vi "ArmPositionControl.vi"(9 "DriverJoystickButtons":bool[](array[boolean]), 10 "ButtonBox2":bool[](array[boolean]), 11 "Buttons":bool[](array[boolean])=[FALSE, FALSE, FALSE, FALSE, FALSE, FALSE, FALSE, FALSE, FALSE, FALSE, FALSE, FALSE]) -> ()   [LabVIEW 2015]
uses:
  Utilities/MotorPositionGlobals.vi
  Utilities/VisionGlobals.vi
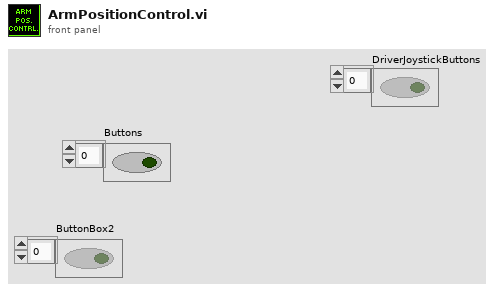
[diagram p1: front panel]
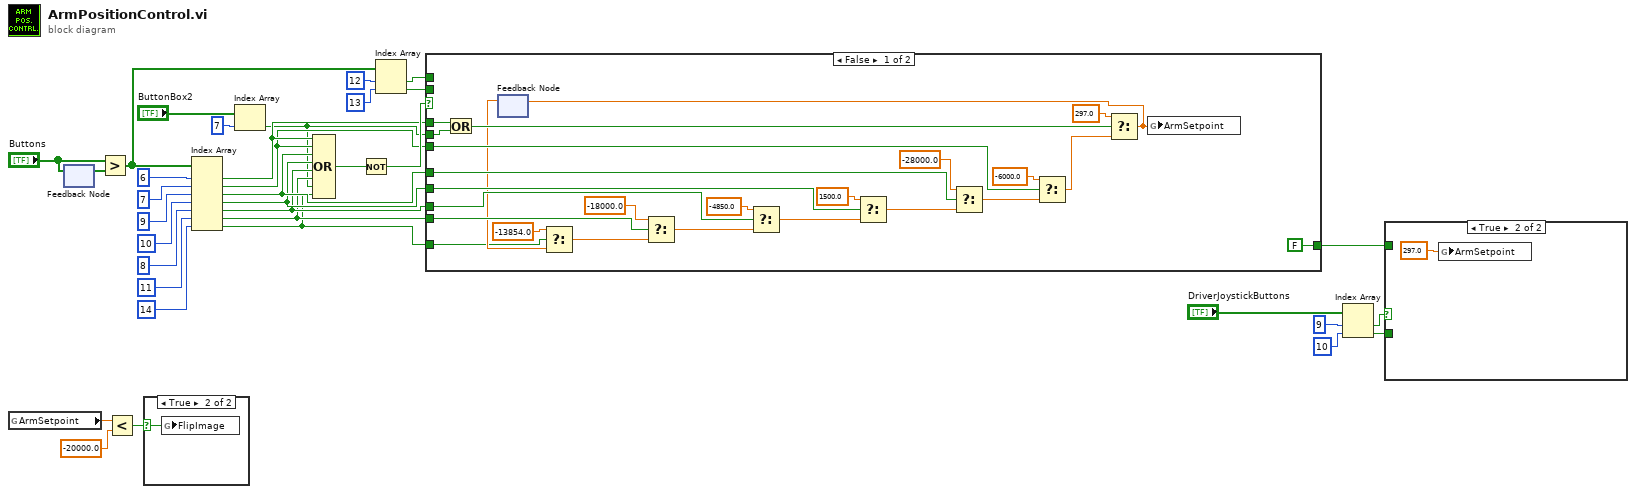
[diagram p0: block diagram]
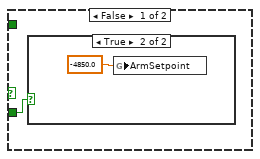
[diagram p2: hidden frame]
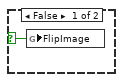
[diagram p4: hidden frame]
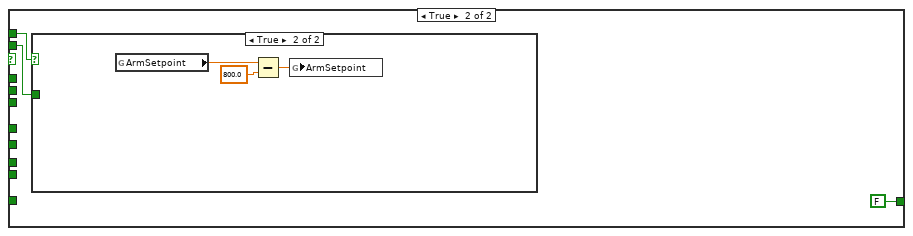
[diagram p5: hidden frame]
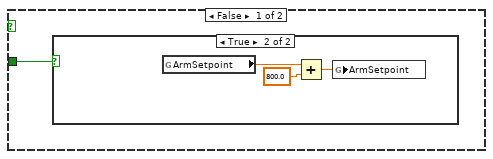
[diagram p6: hidden frame]
diagram:
  n1 = global read "MotorPositionGlobals.vi" "ArmSetpoint"() -> (w20:dbl)
  n2 = feedback-in #1("Buttons") -> ()
  n3 = feedback #1() -> (w32:bool[])  [unwired: 1 in]
  n4 = Greater?(x="Buttons", y=w32) -> (0:w17:bool[])
  n5 = Less?(x=w20, y=-20000.0) -> (x < y?=w18:bool)
  n6 = case shown="True" w18 {
    selector: w18 -> [w36 w37]
    frame False {
      n7 = global write "VisionGlobals.vi" "FlipImage"(w36) -> ()
    }
    frame True {
      n8 = global write "VisionGlobals.vi" "FlipImage"(w37) -> ()
    }
  }
  n9 = Index Array(array=w17, index #1=6 ("index"), index #2=7 ("index"), index #3=9 ("index"), index #4=10 ("index"), index #5=8 ("index"), index #6=11 ("index"), index #7=14 ("index")) -> (element #1=w26:bool, element #2=w25:bool, element #3=w24:bool, element #4=w23:bool, element #5=w21:bool, element #6=w12:bool, element #7=w1:bool)
  n10 = Index Array(array="ButtonBox2", index=7) -> (element=w9:bool)
  n11 = Compound Arithmetic op=OR(w26, w25, w24, w23, w21, w12, w9, w1) -> (w29:bool)
  n12 = Not(x=w29) -> (.not. x?=w28:bool)
  n13 = Index Array(array=w17, index #1=12 ("index"), index #2=13 ("index")) -> (element #1=w15:bool, element #2=w14:bool)
  n14 = case shown="False" w28 {
    tunnel: w26 -> [w44 _]
    tunnel: w25 -> [w55 _]
    tunnel: w23 -> [w54 _]
    tunnel: w24 -> [w53 _]
    tunnel: w21 -> [w51 _]
    tunnel: w15 -> [_ w65]
    tunnel: w14 -> [_ w64]
    tunnel: w12 -> [w47 _]
    tunnel: w9 -> [w45 _]
    tunnel: [FALSE FALSE] -> w8
    tunnel: w1 -> [w39 _]
    frame False {
      n15 = Or(x=w44, y=w45) -> (x .or. y?=w43:bool)
      n16 = feedback #2() -> (w41:dbl)  [unwired: 1 in]
      n17 = Select(t=-13854.0, s=w39, f=w41) -> (s? t:f=w40:dbl)
      n18 = Select(t=-18000.0, s=w47, f=w40) -> (s? t:f=w48:dbl)
      n19 = Select(t=-4850.0, s=w51, f=w48) -> (s? t:f=w50:dbl)
      n20 = Select(t=1500.0 ("t 2"), s=w54, f=w50) -> (s? t:f=w61:dbl)
      n21 = Select(t=-28000.0 ("lower limit"), s=w53, f=w61) -> (s? t:f=w57:dbl)
      n22 = Select(t=-6000.0, s=w55, f=w57) -> (s? t:f=w56:dbl)
      n23 = Select(t=297.0, s=w43, f=w56) -> (s? t:f=w49:dbl)
      n24 = feedback-in #2(w49) -> ()
      n25 = global write "MotorPositionGlobals.vi" "ArmSetpoint"(w49) -> ()
    }
    frame True {
      n26 = case shown="True" w65 {
        tunnel: w64 -> [w66 _]
        frame False {
          n27 = case shown="True" w66 {
            frame False {
            }
            frame True {
              n28 = global read "MotorPositionGlobals.vi" "ArmSetpoint"() -> (w69:dbl)
              n29 = Add(x=w69, y=800.0) -> (x+y=w67:dbl)
              n30 = global write "MotorPositionGlobals.vi" "ArmSetpoint"(w67) -> ()
            }
          }
        }
        frame True {
          n31 = global read "MotorPositionGlobals.vi" "ArmSetpoint"() -> (w72:dbl)
          n32 = Subtract(x=w72, y=800.0) -> (x-y=w70:dbl)
          n33 = global write "MotorPositionGlobals.vi" "ArmSetpoint"(w70) -> ()
        }
      }
    }
  }
  n34 = Index Array(array="DriverJoystickButtons", index #1=9 ("index"), index #2=10 ("index")) -> (element #1=w3:bool, element #2=w5:bool)
  n35 = case shown="True" w3 {
    tunnel: w5 -> [w73 _]
    tunnel: w8 -> [_ _]
    frame False {
      n36 = case shown="True" w73 {
        frame False {
        }
        frame True {
          n37 = global write "MotorPositionGlobals.vi" "ArmSetpoint"(-4850.0 ("ArmSetpoint")) -> ()
        }
      }
    }
    frame True {
      n38 = global write "MotorPositionGlobals.vi" "ArmSetpoint"(297.0 ("ArmSetpoint")) -> ()
    }
  }
